vi "Check Signal Lines.vi"() -> ()   [LabVIEW 2011]
uses:
  <vilib>/rvi/eio/common/nirviEmuTemplateMethod_errors.vi
  <vilib>/eio/EIONode/EIONode.xnode
panel:
  out "Signal":bool[](array[boolean])
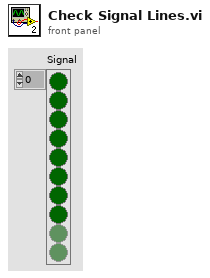
[diagram p1: front panel]
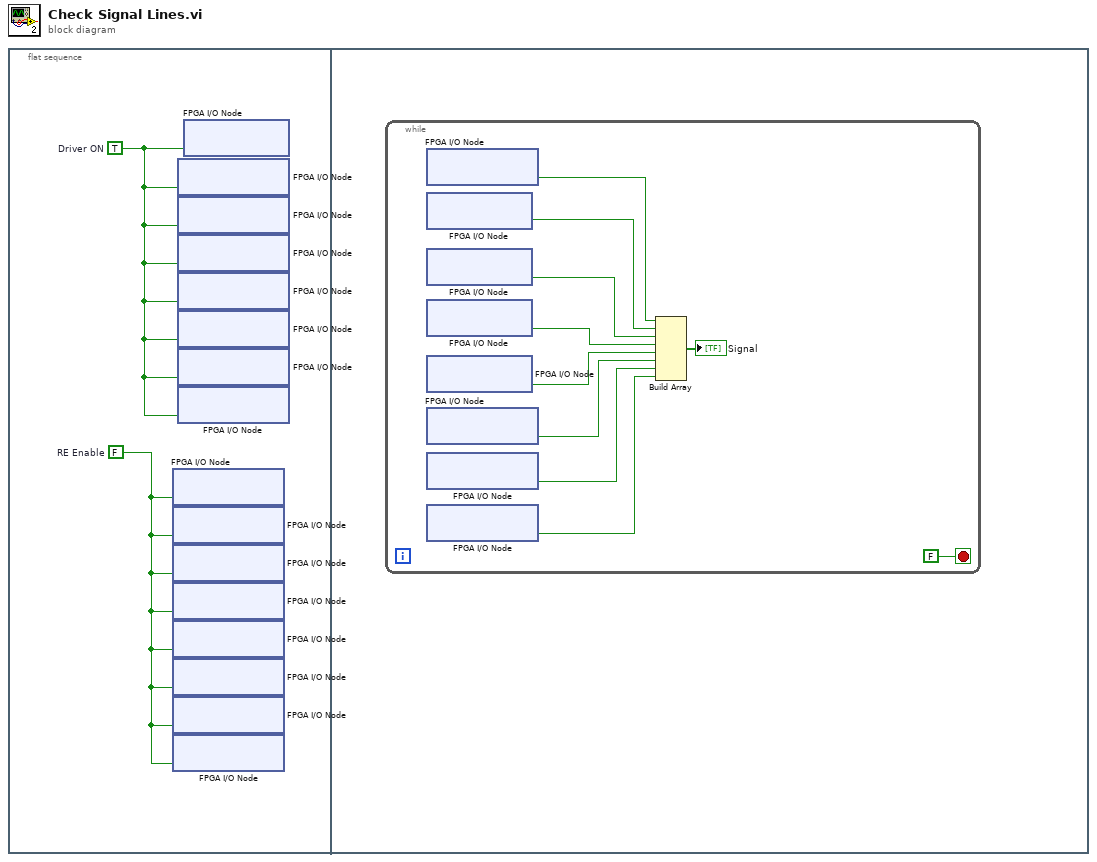
[diagram p0: block diagram]
diagram:
  n1 = flat-sequence {
    frame #0 {
      w1 = TRUE  # Driver ON
      w2 = FALSE  # RE Enable
      n2 = xnode "FPGA I/O Node"("JAGM/DIO32"=w2) -> ()  [unwired: 1 in, 1 out]
      n3 = xnode "FPGA I/O Node"("JAGM/DIO41"=w2) -> ()  [unwired: 1 in, 1 out]
      n4 = xnode "FPGA I/O Node"("JAGM/DIO47"=w2) -> ()  [unwired: 1 in, 1 out]
      n5 = xnode "FPGA I/O Node"("JAGM/DIO54"=w2) -> ()  [unwired: 1 in, 1 out]
      n6 = xnode "FPGA I/O Node"("JAGM/DIO50"=w2) -> ()  [unwired: 1 in, 1 out]
      n7 = xnode "FPGA I/O Node"("JAGM/DIO37"=w2) -> ()  [unwired: 1 in, 1 out]
      n8 = xnode "FPGA I/O Node"("JAGM/DIO45"=w2) -> ()  [unwired: 1 in, 1 out]
      n9 = xnode "FPGA I/O Node"("JAGM/DIO27"=w2) -> ()  [unwired: 1 in, 1 out]
      n10 = xnode "FPGA I/O Node"("JAGM/DIO38"=w1) -> ()  [unwired: 1 in, 1 out]
      n11 = xnode "FPGA I/O Node"("JAGM/DIO15"=w1) -> ()  [unwired: 1 in, 1 out]
      n12 = xnode "FPGA I/O Node"("JAGM/DIO55"=w1) -> ()  [unwired: 1 in, 1 out]
      n13 = xnode "FPGA I/O Node"("JAGM/DIO52"=w1) -> ()  [unwired: 1 in, 1 out]
      n14 = xnode "FPGA I/O Node"("JAGM/DIO35"=w1) -> ()  [unwired: 1 in, 1 out]
      n15 = xnode "FPGA I/O Node"("JAGM/DIO43"=w1) -> ()  [unwired: 1 in, 1 out]
      n16 = xnode "FPGA I/O Node"("JAGM/DIO60"=w1) -> ()  [unwired: 1 in, 1 out]
      n17 = xnode "FPGA I/O Node"("JAGM/DIO0"=w1) -> ()  [unwired: 1 in, 1 out]
    }
    frame #1 {
      n18 = while {
        stop <- FALSE stop-if-true
        n19 = xnode "FPGA I/O Node"() -> ("JAGM/DIO16"=w12:bool)  [unwired: 1 in, 1 out]
        n20 = xnode "FPGA I/O Node"() -> ("JAGM/DIO2"=w11:bool)  [unwired: 1 in, 1 out]
        n21 = xnode "FPGA I/O Node"() -> ("JAGM/DIO4"=w10:bool)  [unwired: 1 in, 1 out]
        n22 = xnode "FPGA I/O Node"() -> ("JAGM/DIO6"=w9:bool)  [unwired: 1 in, 1 out]
        n23 = xnode "FPGA I/O Node"() -> ("JAGM/DIO8"=w8:bool)  [unwired: 1 in, 1 out]
        n24 = xnode "FPGA I/O Node"() -> ("JAGM/DIO10"=w7:bool)  [unwired: 1 in, 1 out]
        n25 = xnode "FPGA I/O Node"() -> ("JAGM/DIO12"=w6:bool)  [unwired: 1 in, 1 out]
        n26 = xnode "FPGA I/O Node"() -> ("JAGM/DIO14"=w5:bool)  [unwired: 1 in, 1 out]
        n27 = Build Array(w12, w11, w10, w9, w8, w7, w6, w5) -> (→"Signal":bool[])
      }
    }
  }
